vi "SubVI_Open_Optimal_Model.vi"(8 "error in (no error)":errorcluster) -> (0 "error out":errorcluster, 4 "Optimal Model Parameters":T1, 6 "Channel_selection":i32[](array[numeric]))   [LabVIEW 2020]
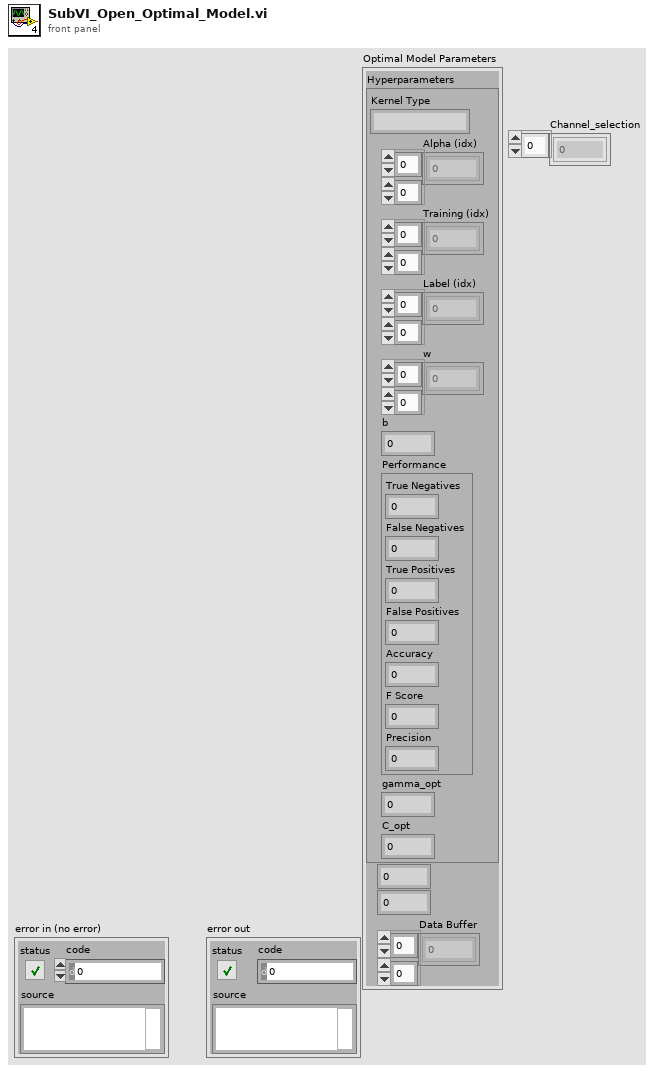
[diagram p1: front panel]
types:
  T1 = cluster{"Hyperparameters":cluster{"Kernel Type":string, "Alpha (idx)":dbl[][], "Training (idx)":dbl[][], "Label (idx)":dbl[][], "w":dbl[][], "b":dbl, "Performance":cluster{"True Negatives":i32, "False Negatives":i32, "True Positives":i32, "False Positives":i32, "Accuracy":dbl, "F Score":dbl, "Precision":dbl}, "gamma_opt":dbl, "C_opt":dbl}, i32, dbl, "Data Buffer":dbl[][]}
  T2 = enum16{"open", "replace", "create", "open or create", "replace or create", "replace or create with confirmation"}
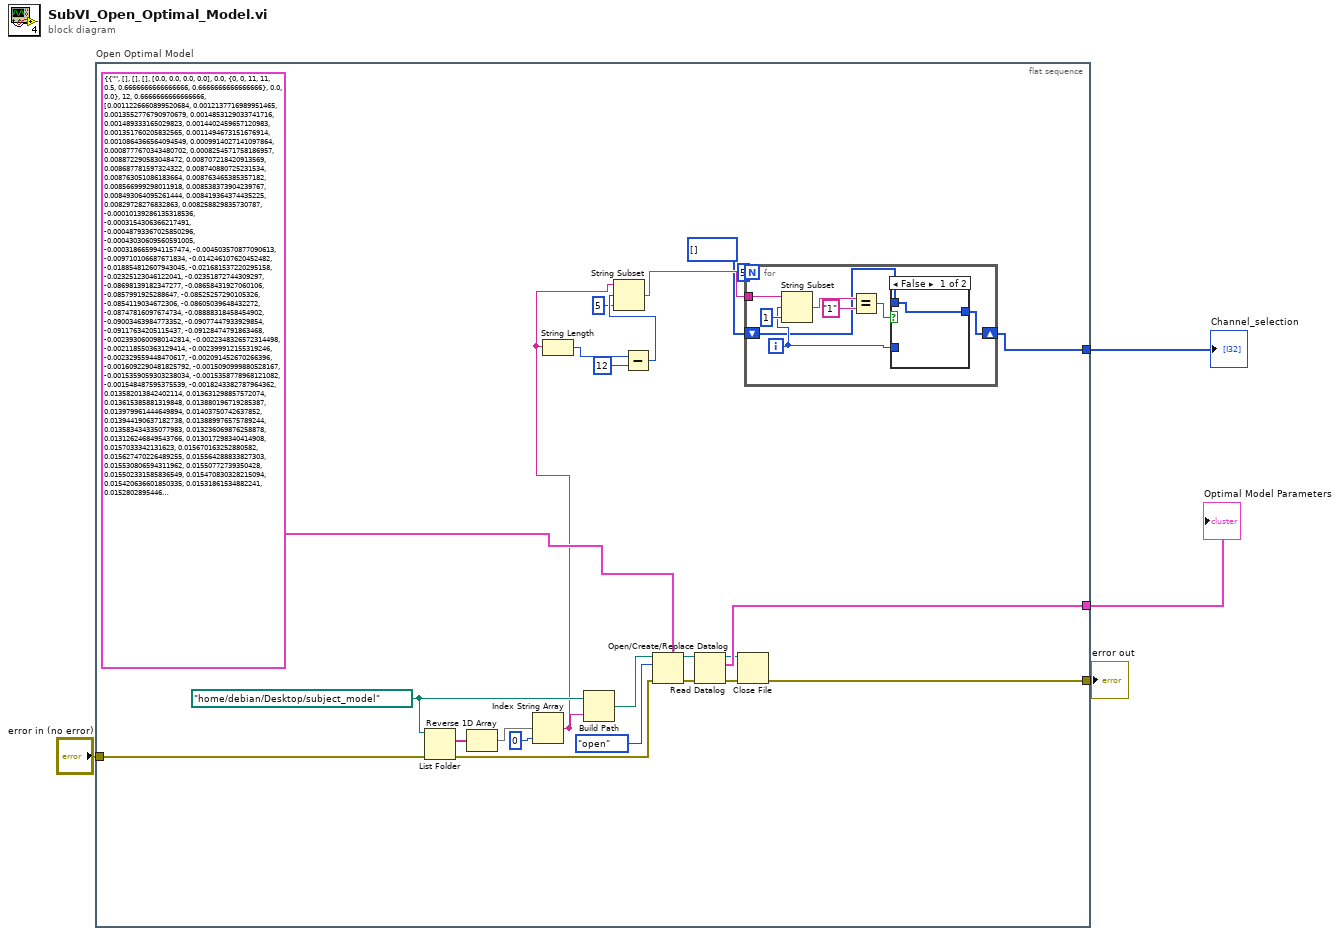
[diagram p0: block diagram]
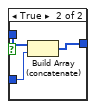
[diagram p2: hidden frame]
diagram:
  n1 = flat-sequence "Open Optimal Model" {
    tunnel: [w28] -> w2
    tunnel: "error in (no error)" -> [w20]
    tunnel: [w22] -> w3
    tunnel: [w5] -> w1
    frame #0 {
      w16 = path "/home/debian/Desktop/subject_model" ("base path")
      n2 = List Folder(path=w16, error in=w20) -> (filenames=w18:string[], error out=w19:errorcluster)  [unwired: 2 in, 2 out]
      n3 = Reverse 1D Array(array=w18) -> (reversed array=w15:string[])
      n4 = Index String Array(1:0 ("index"), 2:w15) -> (0:w9:string)  [unwired: 1 in]
      n5 = String Length(string=w9) -> (length=w13:i32)
      n6 = Build Path(base path=w16, name or relative path=w9) -> (appended path=w26:path)
      n7 = Subtract(x=w13, y=12) -> (x-y=w11:i32)
      n8 = String Subset(string=w9, offset (0)=w11, length (rest)=5 ("length (rest)")) -> (substring=w8:string)
      n9 = Open/Create/Replace Datalog(5:T1 {"Hyperparameters"={"Kernel Type"="", "Alpha (idx)"=[], "Training (idx)"=[], "Label (idx)"=[], "w"=[[0.0], [0.0], [0.0], [0.0]], "b"=0.0, "Performance"={"True Negatives"=0, "False Negatives"=0, "True Positives"=11, "False Positives"=11, "Accuracy"=0.5, "F Score"=0.6666666666666666, "Precision"=0.6666666666666666}, "gamma_opt"=0.0, "C_opt"=0.0}, 12, 0.6666666666666666, "Data Buffer"=[[0.0011226660899520684, 0.0012137716989951465, 0.0013552776790970679, 0.0014853129033741716, 0.001489333165029823, 0.0014402459657120983, 0.001351760205832565, 0.0011494673151676914, 0.0010864366564094549, 0.0009914027141097864, 0.0008777670343480702, 0.0008254571758186957], [0.008872290583048472, 0.008707218420913569, 0.008687781597324322, 0.008740880725231534, 0.008763051086183664, 0.008763465385357182, 0.008566999298011918, 0.008538373904239767, 0.008493064095261444, 0.008419364374435225, 0.00829728276832863, 0.008258829835730787], [-0.00010139286135318536, -0.0003154306366217491, -0.00048793367025850296, -0.00043030609560591005, -0.0003186659941157474, -0.004503570877090613, -0.009710106687671834, -0.014246107620452482, -0.018854812607943045, -0.021681537220295158, -0.02325123046122041, -0.02351872744309297], [-0.08698139182347277, -0.08658431927060106, -0.0857991925288647, -0.08525257290105326, -0.0854119034672306, -0.08605039648432272, -0.08747816097674734, -0.08888318458454902, -0.09003463984773352, -0.09077447933929854, -0.09117634205115437, -0.09128474791863468], [-0.0023930600980142814, -0.0022348326572314498, -0.002118550363129414, -0.002399912155319246, -0.002329559448470617, -0.002091452670266396, -0.0016092290481825792, -0.0015090999880528167, -0.0015359059303238034, -0.0015358778968121082, -0.001548487595375539, -0.0018243382787964362], [0.013582013842402114, 0.013631298857572074, 0.013615385881319848, 0.013880196719285387, 0.013979961444649894, 0.01403750742637852, 0.013944190637182738, 0.013889976575789244, 0.013583434335077983, 0.013236069876258878, 0.013126246849543766, 0.013017298340414908], [0.0157033342131623, 0.015670163252880582, 0.015627470226489255, 0.015564288833827303, 0.015530806594311962, 0.01550772739350428, 0.015502331585836549, 0.015470830328215094, 0.015420636601850335, 0.01531861534882241, 0.015280289544607827, 0.015276157754961193], [0.011828571399811319, 0.011823135524092827, 0.011801121226015185, 0.01180293311638323, 0.011817480781966452, 0.011736448887264488, 0.01165562067678214, 0.011599572343569413, 0.011556704864016464, 0.011523899025902899, 0.011526300550383657, 0.011516670755180878], [0.007888698224376137, 0.007901139861285286, 0.007764442165710794, 0.00771483996331605, 0.007670053479696656, 0.0076056618486329405, 0.007578242800346252, 0.0075829703181126765, 0.007509620379712601, 0.007435755677915998, 0.007301112667225675, 0.007297917652597858], [0.0067902390705444834, 0.006797350258959456, 0.006765177438060157, 0.006789788442956303, 0.006941611219006818, 0.006996363885850453, 0.006866412659615642, 0.006741309468712134, 0.006722252781401622, 0.006689377503446365, 0.006608178325899634, 0.006488238003547652], [0.007799020806841881, 0.007886166798581527, 0.007938224953758111, 0.007995071216758626, 0.008023752238666844, 0.008030068666973061, 0.007874761697119596, 0.007775570905495748, 0.007744913451665303, 0.00765205144221989, 0.0075594522438250265, 0.007503856616890166]]} ("output cluster"), 8:w19, 10:T2."open" ("operation (0:open)"), 11:w26) -> (0:w23:errorcluster, 3:w27:refnum<k1>)  [unwired: 3 out]
      n10 = Read Datalog(4:w23, 7:w27) -> (0:w25:errorcluster, 2:w28:T1, 3:w24:refnum<k1>)  [unwired: 1 in]
      n11 = Close File(refnum=w24, error in=w25) -> (error out=w22:errorcluster)  [unwired: 1 out]
      n12 = for {
        N: 5 -> [_]
        tunnel: w8 -> [w35]
        shift-right: [w30] -> w5
        shift-left: i32[] [] -> [w29]
        i -> [w31]
        n13 = String Subset(string=w35, offset (0)=w31, length (rest)=1 ("length (rest)")) -> (substring=w34:string)
        n14 = Equal?(x=w34, y="1") -> (x = y?=w32:bool)
        n15 = case shown="False" w32 {
          tunnel: w31 -> [_ w40]
          tunnel: [w37 w39] -> w30
          tunnel: w29 -> [w37 w38]
          frame False {
          }
          frame True {
            n16 = Build Array (concatenate)(w38, w40) -> (w39:i32[])
          }
        }
      }
    }
  }
  "error out" <- w3
  "Optimal Model Parameters" <- w2
  "Channel_selection" <- w1
